vi "MSEncoder Act ExportMthd.vi"(8 "error in (no error)":errorcluster, 11 "MSEncoder in":refnum<class "MSEncoder.lvclass">) -> (0 "error out":errorcluster, 2 "Mthd out":T1)   [LabVIEW 2018, in "MSEncoder.lvclass"]
uses:
  MSEncoder.lvclass
  MSEncoder.lvclass/MSEncoder.ctl
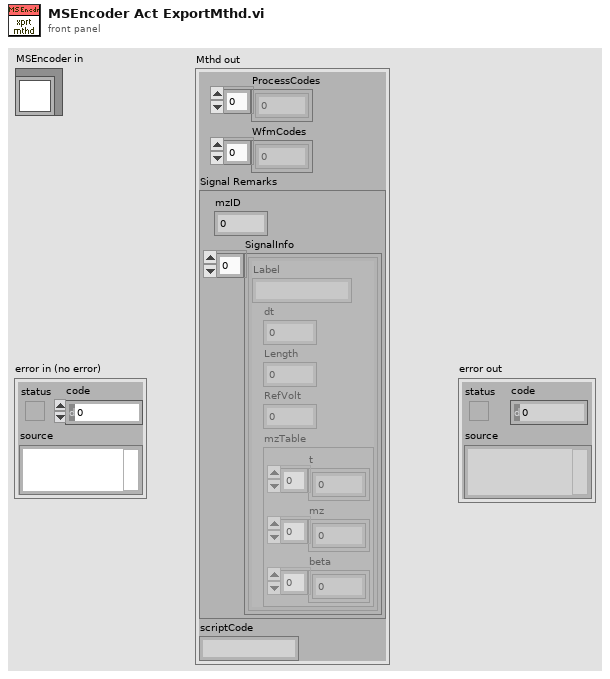
[diagram p1: front panel]
types:
  T1 = cluster{"ProcessCodes":u64[], "WfmCodes":u64[], "Signal Remarks":cluster{"mzID":u64, "SignalInfo":cluster{"Label":string, "dt":dbl, "Length":u32, "RefVolt":dbl, "mzTable":cluster{"t":dbl[], "mz":dbl[], "beta":dbl[]}}[]}, "scriptCode":string}
  T2 = cluster{"mzID":u64, "SignalInfo":cluster{"Label":string, "dt":dbl, "Length":u32, "RefVolt":dbl, "mzTable":cluster{"t":dbl[], "mz":dbl[], "beta":dbl[]}}[]}
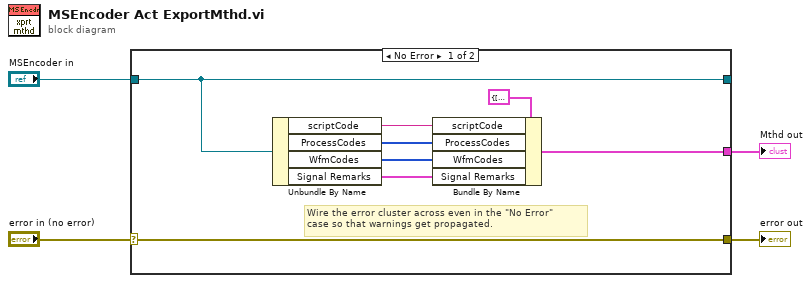
[diagram p0: block diagram]
diagram:
  n1 = case shown="No Error" "error in (no error)" {
    selector: "error in (no error)" -> [w12 w14]
    tunnel: [w12 w14] -> w3
    tunnel: [w11 w13] -> _
    tunnel: "MSEncoder in" -> [w11 w13]
    tunnel: [w7 _] -> w1
    frame No Error {
      # "Wire the error cluster across even in the \"No Error\"\ncase so that warnings get propagated."
      n2 = Unbundle By Name(w11) -> ("scriptCode"=w9:string, "ProcessCodes"=w10:u64[], "WfmCodes"=w8:u64[], "Signal Remarks"=w6:T2)
      n3 = Bundle By Name(cluster=T1 {"ProcessCodes"=[], "WfmCodes"=[], "Signal Remarks"={"mzID"=0, "SignalInfo"=[]}, "scriptCode"=""} ("Mthd out"), "scriptCode"=w9, "ProcessCodes"=w10, "WfmCodes"=w8, "Signal Remarks"=w6) -> (w7:T1)
    }
    frame Error {
    }
  }
  "error out" <- w3
  "Mthd out" <- w1
